vi "ManipHumanPlayerSignal.vi"(11 "Instruction String":string) -> (1 "Error Out":errorcluster, 3 "Advance Trigger":bool)   [LabVIEW 2020]
uses:
  SafeParser_String.vi
  drivercommands.vi
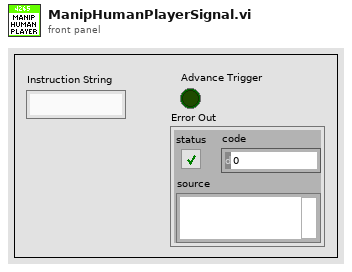
[diagram p1: front panel]
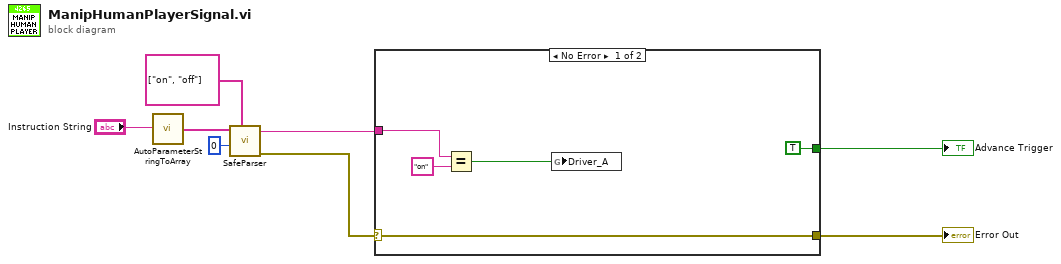
[diagram p0: block diagram]
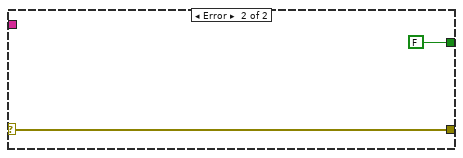
[diagram p2: hidden frame]
diagram:
  n1 = call "AutoParameterStringToArray.vi"("Parameter String"="Instruction String") -> ("Parsed Parameters"=w5:string[])
  n2 = call-poly "SafeParser.vi"("Allowed Values"=string[] ["on", "off"], "Array Index"=0 ("Parameter Index"), "String Array"=w5) -> ("Error Out"=w3:errorcluster, "Typecast Value"=w4:string)  [unwired: 7 in]
  n3 = case shown="No Error" w3 {
    selector: w3 -> [w12 w14]
    tunnel: [TRUE ("Advance Trigger") FALSE ("Advance Trigger")] -> w8
    tunnel: [w12 w14] -> w7
    tunnel: w4 -> [w11 _]
    frame No Error {
      n4 = Equal?(x=w11, y="on") -> (x = y?=w10:bool)
      n5 = global write "drivercommands.vi" "Driver_A"(w10) -> ()
    }
    frame Error {
    }
  }
  "Advance Trigger" <- w8
  "Error Out" <- w7
